vi "Get All Channel Data.vi"(8 "Original T0":timestamp, 9 "waveform in":waveform(dbl), 10 "TDMS Channel Info":T1, 11 "CSV Settings":T2={"Log Stats"=FALSE, "Time Format"="%H:%M:%S%3u", "Resampled"=FALSE, "Resampled Rate"=0.0, "Digits of Precision"=0, "Relative Time"=FALSE, "Log Units"=FALSE, "Log Properties"=FALSE}) -> (3 "String Data":string[](array[string]))   [LabVIEW 2022 SP3, in "CSV Export.lvlib" / "CSV Export.lvclass"]
uses:
  CSV Export.lvclass
  Controls/CSV Export Settings.ctl
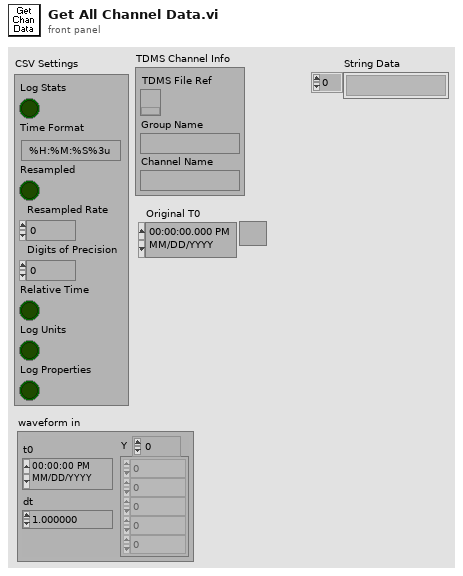
[diagram p1: front panel]
types:
  T1 = cluster{"TDMS File Ref":refnum<k34>, "Group Name":string, "Channel Name":string}
  T2 = typedef "CSV Export.lvlib/CSV Export.lvclass/CSV Export Settings.ctl" = cluster{"Log Stats":bool, "Time Format":string, "Resampled":bool, "Resampled Rate":dbl, "Digits of Precision":u32, "Relative Time":bool, "Log Units":bool, "Log Properties":bool}
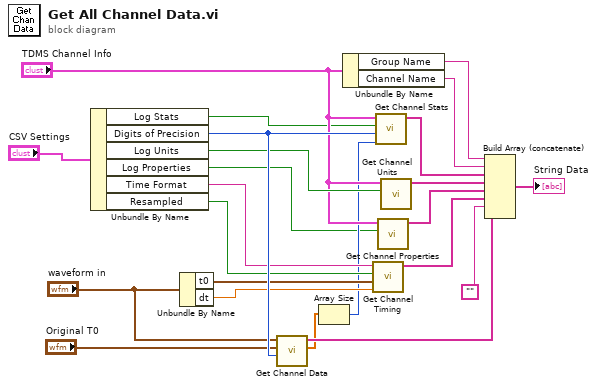
[diagram p0: block diagram]
diagram:
  n1 = Unbundle By Name("CSV Settings") -> ("Log Stats"=w2:bool, "Digits of Precision"=w22:u32, "Log Units"=w9:bool, "Log Properties"=w1:bool, "Time Format"=w10:string, "Resampled"=w11:bool)
  n2 = Unbundle By Name("waveform in") -> ("t0"=w17:timestamp, "dt"=w16:dbl)
  n3 = call "Get Channel Data.vi"("Digits of Precision"=w22, "Original T0"="Original T0", "waveform in"="waveform in") -> ("Corrected Data"=w7:dbl[], "Resulting Data String"=w20:string[])  [unwired: 7 in]
  n4 = Array Size(array=w7) -> (size(s)=w6:i32)
  n5 = Unbundle By Name("TDMS Channel Info") -> ("Group Name"=w5:string, "Channel Name"=w4:string)
  n6 = call "Get Channel Timing.vi"("dt"=w16, "T0"=w17, "Resample"=w11, "Time Format"=w10) -> ("Channel Stats"=w13:string[])  [unwired: 7 in]
  n7 = call "Get Channel Stats.vi"("Array Length"=w6, "Number of Precision Digits"=w22, "Log Stats"=w2, "TDMS Channel Info"="TDMS Channel Info") -> ("Channel Stats"=w3:string[])  [unwired: 7 in]
  n8 = call "Get Channel Properties.vi"("Log Properties"=w1, "TDMS Channel Info"="TDMS Channel Info") -> ("Property String Out"=w12:string[])  [unwired: 9 in]
  n9 = call "Get Channel Units.vi"("Log Units"=w9, "TDMS Channel Info"="TDMS Channel Info") -> ("Unit String Out"=w14:string[])  [unwired: 9 in]
  n10 = Build Array (concatenate)(w5, w4, w3, w14, w12, w13, "", w20) -> (→"String Data":string[])
